vi "PC_HMI_Lift.vi"() -> ()   [LabVIEW 2014]
panel:
  out "Boolean 12":bool
  out "Boolean 11":bool
  out "Boolean 10":bool
  out "Boolean 9":bool
  out "Boolean 8":bool
  out "Boolean 7":bool
  out "Boolean 6":bool
  out "Boolean 5":bool
  out "Boolean 4":bool
  out "Boolean 3":bool
  out "Boolean 2":bool
  out "Boolean":bool
  out "6":bool
  out "4":bool
  out "5":bool
  out "3":bool
  out "2":bool
  out "1":bool
  out "0":bool
  in  "STOP":bool
  in  "SPRAT 5":bool
  in  "SPRAT 4":bool
  in  "SPRAT 3":bool
  in  "SPRAT 2":bool
  in  "SPRAT 1":bool
  in  "SPRAT 0":bool
  out "IDLE":bool
  out "SHUTDOWN":bool
  out "MOVING":bool
  out "DOOR OPEN":bool
  in  "GORE 4":bool
  in  "DOLE 4":bool
  in  "DOLE 5":bool
  in  "GORE 3":bool
  in  "DOLE 3":bool
  in  "GORE 2":bool
  in  "DOLE 2":bool
  in  "GORE 1":bool
  in  "DOLE 1":bool
  in  "GORE 0":bool
  out "Meter":dbl(knob) scale=0.0..5.0
  out "x":dbl
  out "GRAFIK":dbl(graph)
  out "u":dbl
  # "SPRAT 5"
  # "SPRAT 4"
  # "SPRAT 3"
  # "SPRAT 2"
  # "SPRAT 1"
  # "PRIZEMLJE"
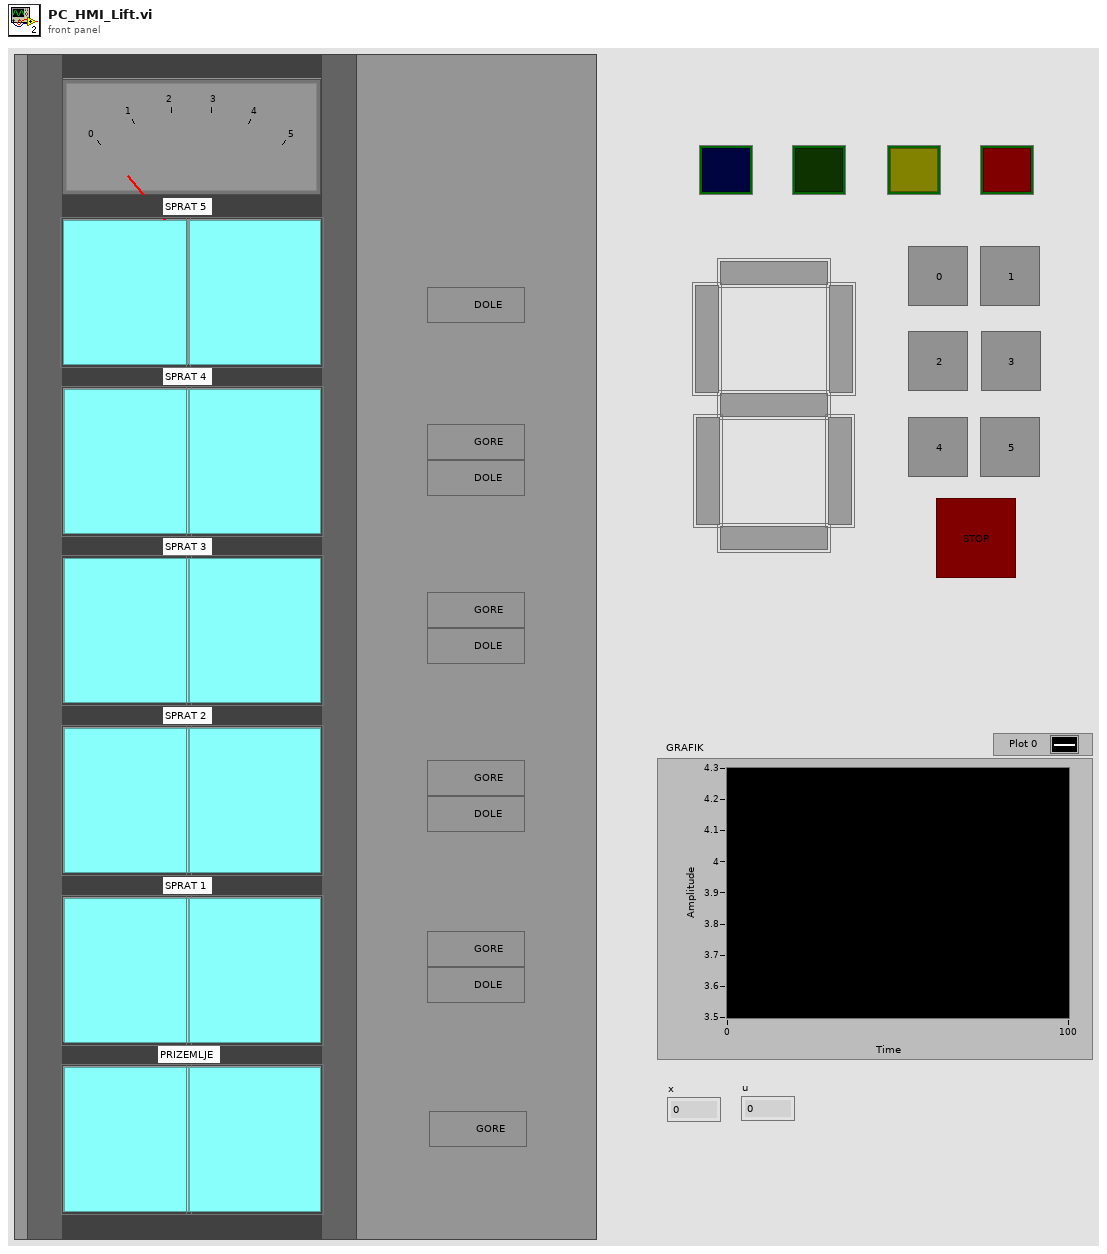
[diagram p1: front panel]
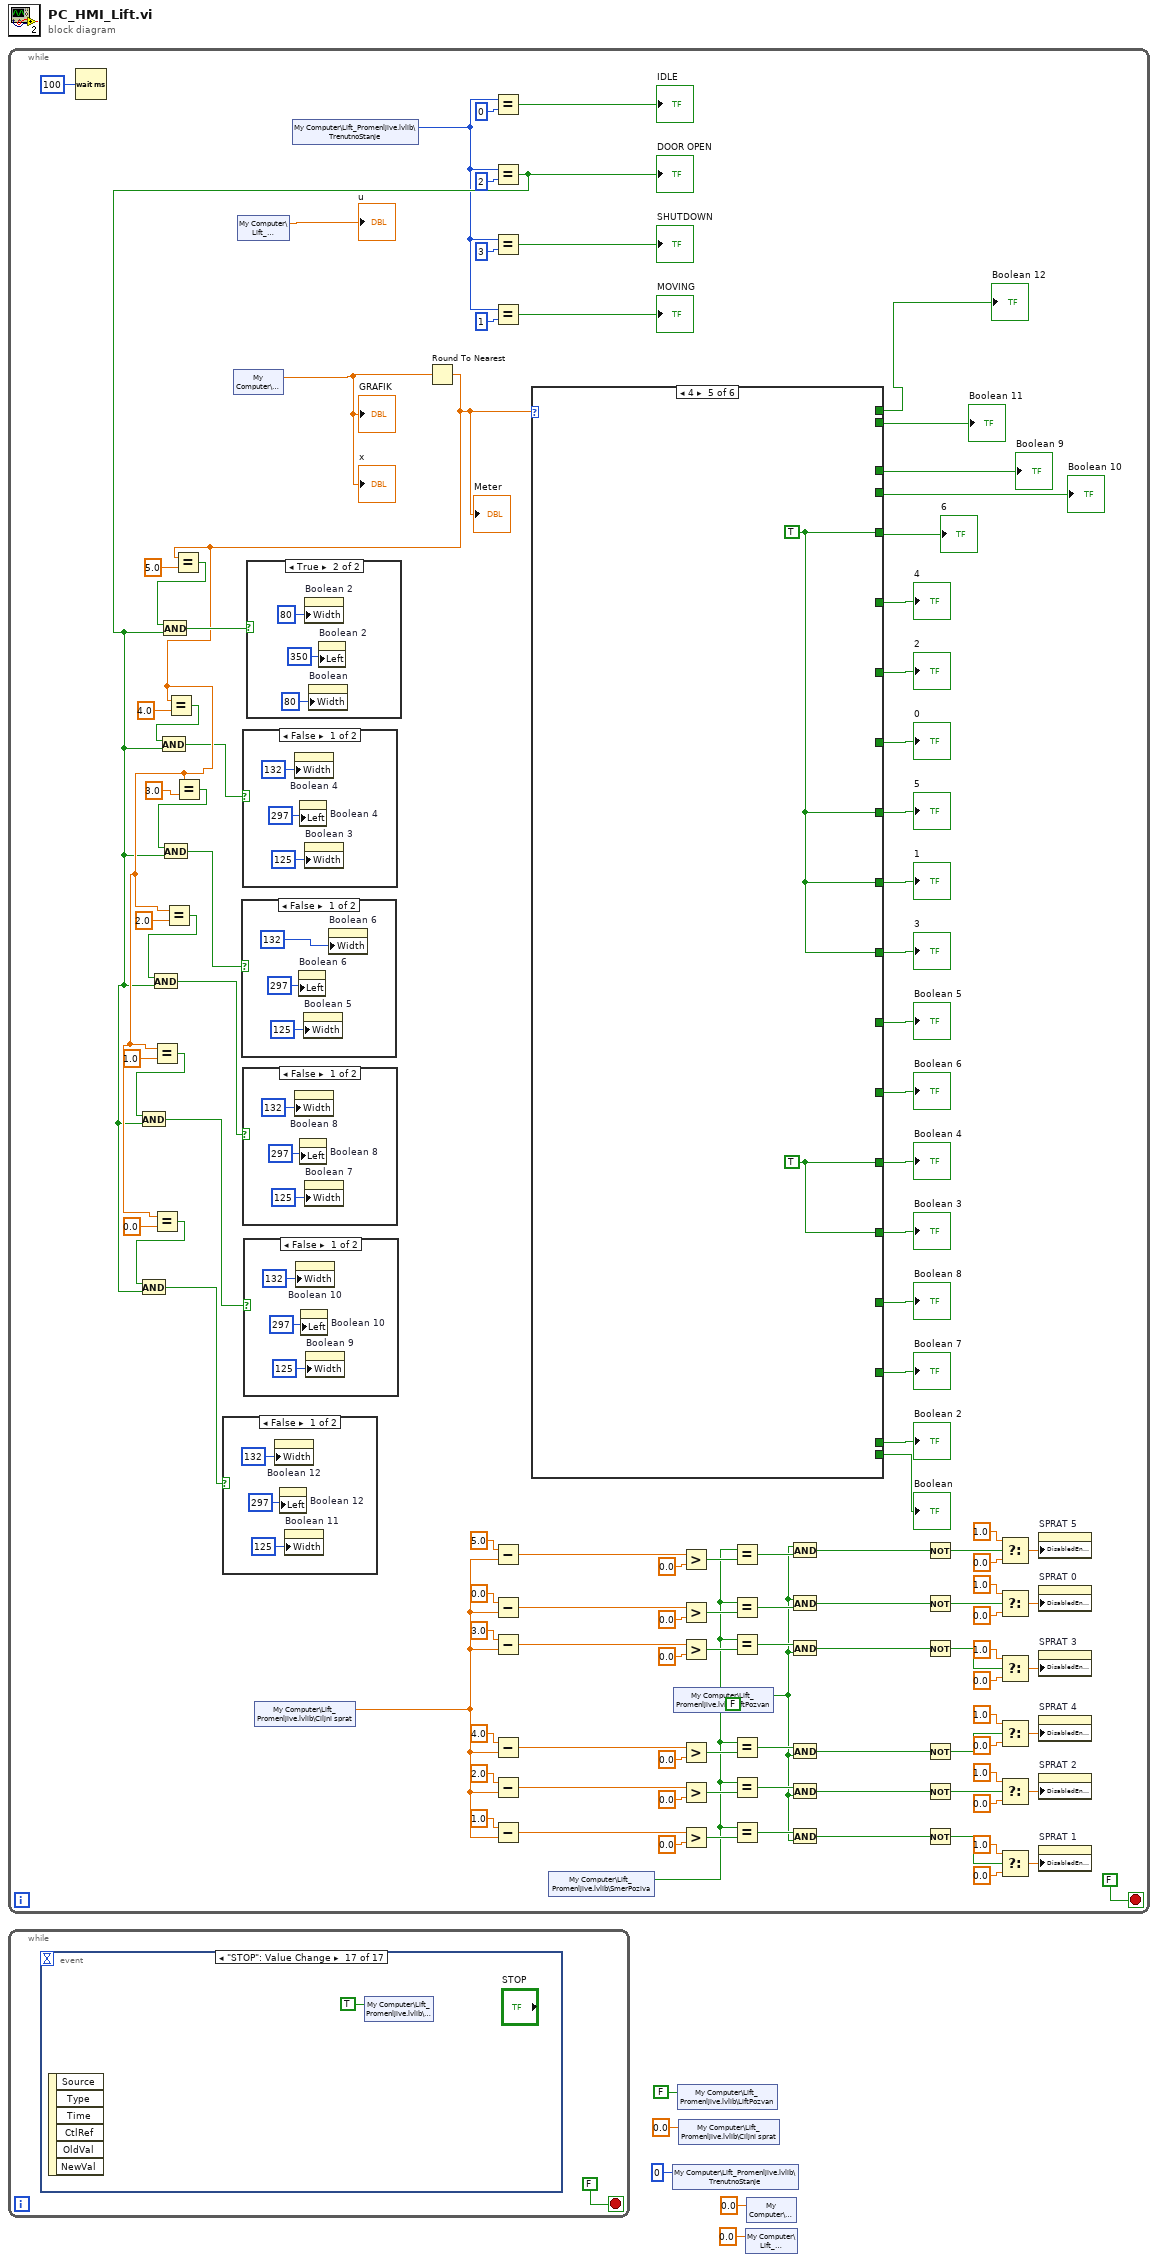
[diagram p0: block diagram]
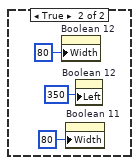
[diagram p2: hidden frame]
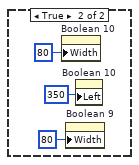
[diagram p3: hidden frame]
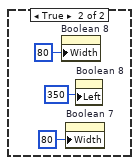
[diagram p4: hidden frame]
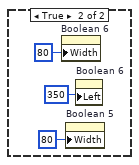
[diagram p5: hidden frame]
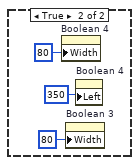
[diagram p6: hidden frame]
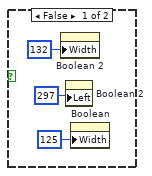
[diagram p7: hidden frame]
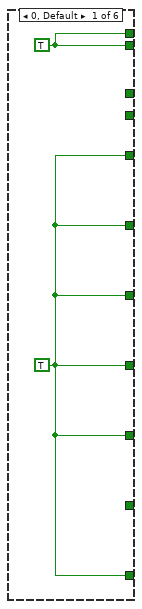
[diagram p8: hidden frame]
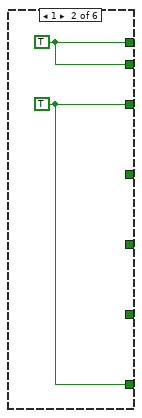
[diagram p9: hidden frame]
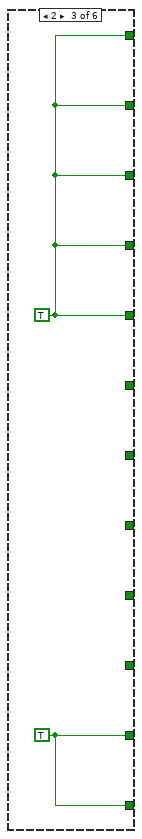
[diagram p10: hidden frame]
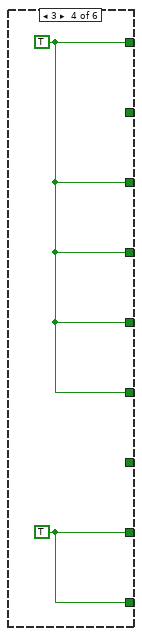
[diagram p11: hidden frame]
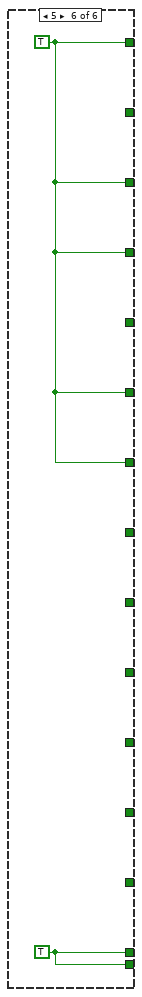
[diagram p12: hidden frame]
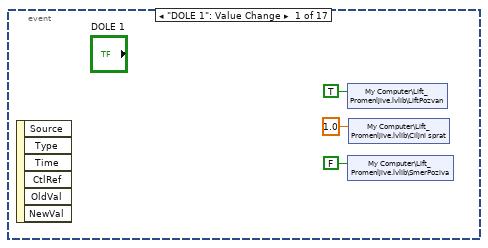
[diagram p13: hidden frame]
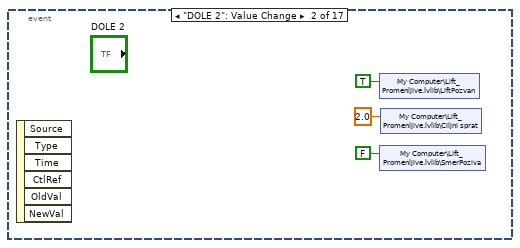
[diagram p14: hidden frame]
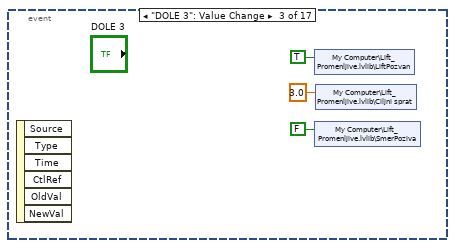
[diagram p15: hidden frame]
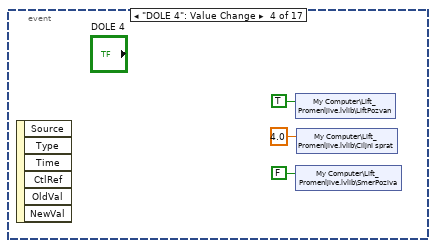
[diagram p16: hidden frame]
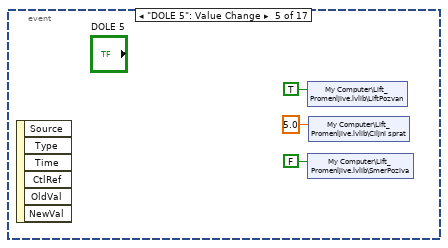
[diagram p17: hidden frame]
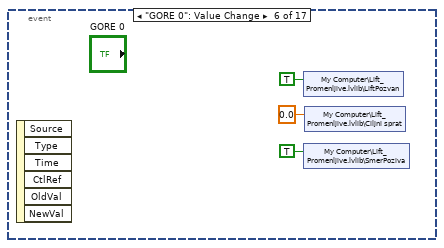
[diagram p18: hidden frame]
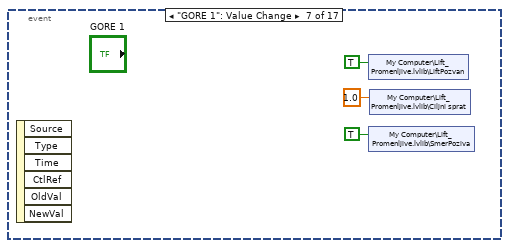
[diagram p19: hidden frame]
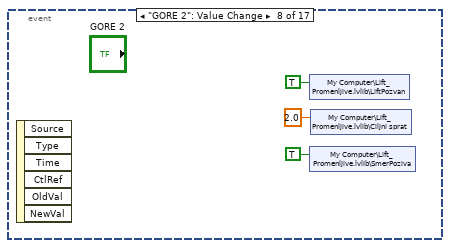
[diagram p20: hidden frame]
diagram:
  n1 = while {
    stop <- FALSE stop-if-true
    (unwired) FALSE
    n2 = Wait (ms)(milliseconds to wait=u32 100) -> ()  [unwired: 1 out]
    n3 = shared-variable "My Computer\\Lift_Promenljive.lvlib\\x"() -> (w9:dbl)  [unwired: 1 in, 1 out]
    "x" <- w9
    "GRAFIK" <- w9
    n4 = shared-variable "My Computer\\Lift_Promenljive.lvlib\\u"() -> (→"u":dbl)  [unwired: 1 in, 1 out]
    n5 = shared-variable "My Computer\\Lift_Promenljive.lvlib\\Ciljni sprat"() -> (w7:dbl)  [unwired: 1 in, 1 out]
    n6 = shared-variable "My Computer\\Lift_Promenljive.lvlib\\TrenutnoStanje"() -> (w11:u8)  [unwired: 1 in, 1 out]
    n7 = Round To Nearest(number=w9) -> (nearest integer value=w18:dbl)
    "Meter" <- w18
    n8 = Equal?(x=w18, y=1.0) -> (x = y?=w21:bool)
    n9 = Equal?(x=w18, y=0.0) -> (x = y?=w19:bool)
    n10 = Equal?(x=w18, y=2.0) -> (x = y?=w23:bool)
    n11 = Equal?(x=w18, y=4.0) -> (x = y?=w27:bool)
    n12 = Equal?(x=w18, y=5.0) -> (x = y?=w30:bool)
    n13 = Equal?(x=w18, y=3.0) -> (x = y?=w25:bool)
    n14 = Equal?(x=w11, y=0) -> (x = y?=→"IDLE":bool)
    n15 = Equal?(x=w11, y=2) -> (x = y?=w17:bool)
    "DOOR OPEN" <- w17
    n16 = And(x=w21, y=w17) -> (x .and. y?=w15:bool)
    n17 = And(x=w19, y=w17) -> (x .and. y?=w16:bool)
    n18 = And(x=w23, y=w17) -> (x .and. y?=w14:bool)
    n19 = And(x=w27, y=w17) -> (x .and. y?=w12:bool)
    n20 = And(x=w30, y=w17) -> (x .and. y?=w29:bool)
    n21 = And(x=w25, y=w17) -> (x .and. y?=w13:bool)
    n22 = case shown="False" w16 {
      frame False {
        n23 = property on="Boolean 12" class="Bool (strict)"("Width"=u32 132 ("Button Size:Width")) -> ()  [unwired: 2 in, 2 out]
        n24 = property on="Boolean 12" class="Bool (strict)"("Left"=297 ("Position:Left")) -> ()  [unwired: 2 in, 2 out]
        n25 = property on="Boolean 11" class="Bool (strict)"("Width"=u32 125 ("Button Size:Width")) -> ()  [unwired: 2 in, 2 out]
      }
      frame True {
        n26 = property on="Boolean 12" class="Bool (strict)"("Width"=u32 80 ("Button Size:Width")) -> ()  [unwired: 2 in, 2 out]
        n27 = property on="Boolean 11" class="Bool (strict)"("Width"=u32 80 ("Button Size:Width")) -> ()  [unwired: 2 in, 2 out]
        n28 = property on="Boolean 12" class="Bool (strict)"("Left"=350 ("Position:Left")) -> ()  [unwired: 2 in, 2 out]
      }
    }
    n29 = case shown="False" w13 {
      frame False {
        n30 = property on="Boolean 6" class="Bool (strict)"("Left"=297 ("Position:Left")) -> ()  [unwired: 2 in, 2 out]
        n31 = property on="Boolean 5" class="Bool (strict)"("Width"=u32 125 ("Button Size:Width")) -> ()  [unwired: 2 in, 2 out]
        n32 = property on="Boolean 6" class="Bool (strict)"("Width"=u32 132 ("Button Size:Width")) -> ()  [unwired: 2 in, 2 out]
      }
      frame True {
        n33 = property on="Boolean 6" class="Bool (strict)"("Width"=u32 80 ("Button Size:Width")) -> ()  [unwired: 2 in, 2 out]
        n34 = property on="Boolean 5" class="Bool (strict)"("Width"=u32 80 ("Button Size:Width")) -> ()  [unwired: 2 in, 2 out]
        n35 = property on="Boolean 6" class="Bool (strict)"("Left"=350 ("Position:Left")) -> ()  [unwired: 2 in, 2 out]
      }
    }
    n36 = case shown="False" w12 {
      frame False {
        n37 = property on="Boolean 4" class="Bool (strict)"("Width"=u32 132 ("Button Size:Width")) -> ()  [unwired: 2 in, 2 out]
        n38 = property on="Boolean 4" class="Bool (strict)"("Left"=297 ("Position:Left")) -> ()  [unwired: 2 in, 2 out]
        n39 = property on="Boolean 3" class="Bool (strict)"("Width"=u32 125 ("Button Size:Width")) -> ()  [unwired: 2 in, 2 out]
      }
      frame True {
        n40 = property on="Boolean 4" class="Bool (strict)"("Width"=u32 80 ("Button Size:Width")) -> ()  [unwired: 2 in, 2 out]
        n41 = property on="Boolean 3" class="Bool (strict)"("Width"=u32 80 ("Button Size:Width")) -> ()  [unwired: 2 in, 2 out]
        n42 = property on="Boolean 4" class="Bool (strict)"("Left"=350 ("Position:Left")) -> ()  [unwired: 2 in, 2 out]
      }
    }
    n43 = case shown="False" w14 {
      frame False {
        n44 = property on="Boolean 8" class="Bool (strict)"("Width"=u32 132 ("Button Size:Width")) -> ()  [unwired: 2 in, 2 out]
        n45 = property on="Boolean 8" class="Bool (strict)"("Left"=297 ("Position:Left")) -> ()  [unwired: 2 in, 2 out]
        n46 = property on="Boolean 7" class="Bool (strict)"("Width"=u32 125 ("Button Size:Width")) -> ()  [unwired: 2 in, 2 out]
      }
      frame True {
        n47 = property on="Boolean 8" class="Bool (strict)"("Width"=u32 80 ("Button Size:Width")) -> ()  [unwired: 2 in, 2 out]
        n48 = property on="Boolean 7" class="Bool (strict)"("Width"=u32 80 ("Button Size:Width")) -> ()  [unwired: 2 in, 2 out]
        n49 = property on="Boolean 8" class="Bool (strict)"("Left"=350 ("Position:Left")) -> ()  [unwired: 2 in, 2 out]
      }
    }
    n50 = case shown="False" w15 {
      frame False {
        n51 = property on="Boolean 10" class="Bool (strict)"("Width"=u32 132 ("Button Size:Width")) -> ()  [unwired: 2 in, 2 out]
        n52 = property on="Boolean 10" class="Bool (strict)"("Left"=297 ("Position:Left")) -> ()  [unwired: 2 in, 2 out]
        n53 = property on="Boolean 9" class="Bool (strict)"("Width"=u32 125 ("Button Size:Width")) -> ()  [unwired: 2 in, 2 out]
      }
      frame True {
        n54 = property on="Boolean 10" class="Bool (strict)"("Width"=u32 80 ("Button Size:Width")) -> ()  [unwired: 2 in, 2 out]
        n55 = property on="Boolean 9" class="Bool (strict)"("Width"=u32 80 ("Button Size:Width")) -> ()  [unwired: 2 in, 2 out]
        n56 = property on="Boolean 10" class="Bool (strict)"("Left"=350 ("Position:Left")) -> ()  [unwired: 2 in, 2 out]
      }
    }
    n57 = case shown="True" w29 {
      frame False {
        n58 = property on="Boolean 2" class="Bool (strict)"("Width"=u32 132 ("Button Size:Width")) -> ()  [unwired: 2 in, 2 out]
        n59 = property on="Boolean 2" class="Bool (strict)"("Left"=297 ("Position:Left")) -> ()  [unwired: 2 in, 2 out]
        n60 = property on="Boolean" class="Bool (strict)"("Width"=u32 125 ("Button Size:Width")) -> ()  [unwired: 2 in, 2 out]
      }
      frame True {
        n61 = property on="Boolean 2" class="Bool (strict)"("Width"=u32 80 ("Button Size:Width")) -> ()  [unwired: 2 in, 2 out]
        n62 = property on="Boolean" class="Bool (strict)"("Width"=u32 80 ("Button Size:Width")) -> ()  [unwired: 2 in, 2 out]
        n63 = property on="Boolean 2" class="Bool (strict)"("Left"=350 ("Position:Left")) -> ()  [unwired: 2 in, 2 out]
      }
    }
    n64 = Equal?(x=w11, y=3) -> (x = y?=→"SHUTDOWN":bool)
    n65 = Equal?(x=w11, y=1) -> (x = y?=→"MOVING":bool)
    n66 = Subtract(x=5.0, y=w7) -> (x-y=w59:dbl)
    n67 = Subtract(x=0.0 ("y"), y=w7) -> (x-y=w68:dbl)
    n68 = Subtract(x=3.0 ("y"), y=w7) -> (x-y=w100:dbl)
    n69 = Subtract(x=4.0 ("y"), y=w7) -> (x-y=w99:dbl)
    n70 = Subtract(x=2.0 ("y"), y=w7) -> (x-y=w101:dbl)
    n71 = Subtract(x=1.0 ("y"), y=w7) -> (x-y=w105:dbl)
    n72 = case shown="4" w18 {
      tunnel: [w157 _ w161 w163 _ w167] -> w32
      tunnel: [_ _ w161 w163 w165 w167] -> w33
      tunnel: [w157 _ w161 w163 _ w167] -> w34
      tunnel: [w157 _ _ _ w165 w167] -> w35
      tunnel: [w157 _ w161 _ _ _] -> w36
      tunnel: [w157 w159 _ w163 w165 w167] -> w37
      tunnel: [w157 w159 w161 w163 w165 _] -> w38
      tunnel: [w156 _ _ _ _ _] -> w39
      tunnel: [w156 _ _ _ _ _] -> w40
      tunnel: [_ w158 _ _ _ _] -> w41
      tunnel: [_ w158 _ _ _ _] -> w42
      tunnel: [_ _ w160 _ _ _] -> w43
      tunnel: [_ _ w160 _ _ _] -> w44
      tunnel: [_ _ _ w162 _ _] -> w45
      tunnel: [_ _ _ w162 _ _] -> w46
      tunnel: [_ _ _ _ w164 _] -> w47
      tunnel: [_ _ _ _ w164 _] -> w48
      tunnel: [_ _ _ _ _ w166] -> w49
      tunnel: [_ _ _ _ _ w166] -> w50
      frame 0, Default {
        w156 = TRUE
        w157 = TRUE
      }
      frame 1 {
        w158 = TRUE
        w159 = TRUE
      }
      frame 2 {
        w160 = TRUE
        w161 = TRUE
      }
      frame 3 {
        w162 = TRUE
        w163 = TRUE
      }
      frame 4 {
        w164 = TRUE
        w165 = TRUE
      }
      frame 5 {
        w166 = TRUE
        w167 = TRUE
      }
    }
    "1" <- w33
    "2" <- w34
    "3" <- w35
    "5" <- w38
    "4" <- w36
    "6" <- w37
    "0" <- w32
    "Boolean 2" <- w50
    "Boolean" <- w49
    "Boolean 3" <- w48
    "Boolean 4" <- w47
    "Boolean 5" <- w45
    "Boolean 7" <- w43
    "Boolean 6" <- w46
    "Boolean 12" <- w40
    "Boolean 8" <- w44
    "Boolean 10" <- w42
    "Boolean 9" <- w41
    "Boolean 11" <- w39
    n73 = shared-variable "My Computer\\Lift_Promenljive.lvlib\\SmerPoziva"() -> (w6:bool)  [unwired: 1 in, 1 out]
    n74 = shared-variable "My Computer\\Lift_Promenljive.lvlib\\LiftPozvan"() -> (w8:bool)  [unwired: 1 in, 1 out]
    n75 = Greater?(x=w59, y=0.0) -> (0:w57:bool)
    n76 = Greater?(x=w68, y=0.0) -> (0:w67:bool)
    n77 = Greater?(x=w100, y=0.0) -> (0:w96:bool)
    n78 = Greater?(x=w99, y=0.0) -> (0:w95:bool)
    n79 = Greater?(x=w101, y=0.0) -> (0:w97:bool)
    n80 = Greater?(x=w105, y=0.0) -> (0:w98:bool)
    n81 = Equal?(x=w6, y=w57) -> (x = y?=w56:bool)
    n82 = Equal?(x=w6, y=w67) -> (x = y?=w66:bool)
    n83 = Equal?(x=w6, y=w96) -> (x = y?=w92:bool)
    n84 = Equal?(x=w6, y=w95) -> (x = y?=w91:bool)
    n85 = Equal?(x=w6, y=w97) -> (x = y?=w93:bool)
    n86 = Equal?(x=w6, y=w98) -> (x = y?=w94:bool)
    n87 = And(x=w8, y=w56) -> (x .and. y?=w55:bool)
    n88 = And(x=w8, y=w66) -> (x .and. y?=w65:bool)
    n89 = And(x=w92, y=w8) -> (x .and. y?=w88:bool)
    n90 = And(x=w91, y=w8) -> (x .and. y?=w87:bool)
    n91 = And(x=w93, y=w8) -> (x .and. y?=w89:bool)
    n92 = And(x=w94, y=w8) -> (x .and. y?=w90:bool)
    n93 = Not(x=w55) -> (.not. x?=w52:bool)
    n94 = Not(x=w65) -> (.not. x?=w62:bool)
    n95 = Not(x=w88) -> (.not. x?=w75:bool)
    n96 = Not(x=w87) -> (.not. x?=w74:bool)
    n97 = Not(x=w89) -> (.not. x?=w76:bool)
    n98 = Not(x=w90) -> (.not. x?=w86:bool)
    n99 = Select(t=1.0, s=w52, f=0.0) -> (s? t:f=w51:dbl)
    n100 = Select(t=1.0, s=w62, f=0.0) -> (s? t:f=w61:dbl)
    n101 = Select(t=1.0, s=w75, f=0.0) -> (s? t:f=w72:dbl)
    n102 = Select(t=1.0, s=w74, f=0.0) -> (s? t:f=w71:dbl)
    n103 = Select(t=1.0, s=w76, f=0.0) -> (s? t:f=w73:dbl)
    n104 = Select(t=1.0, s=w86, f=0.0) -> (s? t:f=w83:dbl)
    n105 = property on="SPRAT 5" class="Bool"("DisabledEnum"=w51) -> ()  [unwired: 2 in, 2 out]
    n106 = property on="SPRAT 0" class="Bool"("DisabledEnum"=w61) -> ()  [unwired: 2 in, 2 out]
    n107 = property on="SPRAT 3" class="Bool"("DisabledEnum"=w72) -> ()  [unwired: 2 in, 2 out]
    n108 = property on="SPRAT 4" class="Bool"("DisabledEnum"=w71) -> ()  [unwired: 2 in, 2 out]
    n109 = property on="SPRAT 2" class="Bool"("DisabledEnum"=w73) -> ()  [unwired: 2 in, 2 out]
    n110 = property on="SPRAT 1" class="Bool"("DisabledEnum"=w83) -> ()  [unwired: 2 in, 2 out]
  }
  n111 = while {
    stop <- FALSE stop-if-true
    n112 = event shown="[16] \"STOP\": Value Change" {
      selector: _ -> [_ _ _ _ _ _ _ _ _ _ _ _ _ _ _ _ _]
      dyn-events: _ -> [_ _ _ _ _ _ _ _ _ _ _ _ _ _ _ _ _]
      timeout: _ -> [_ _ _ _ _ _ _ _ _ _ _ _ _ _ _ _ _]
      event "DOLE 1": Value Change {
        n113 = event-data() -> ()  [unwired: 1 in, 6 out]
        n114 = shared-variable "My Computer\\Lift_Promenljive.lvlib\\LiftPozvan"(TRUE ("LiftPozvan")) -> ()  [unwired: 1 in, 1 out]
        n115 = shared-variable "My Computer\\Lift_Promenljive.lvlib\\SmerPoziva"(FALSE ("SmerPoziva")) -> ()  [unwired: 1 in, 1 out]
        n116 = shared-variable "My Computer\\Lift_Promenljive.lvlib\\Ciljni sprat"(1.0 ("Ciljni sprat")) -> ()  [unwired: 1 in, 1 out]
      }
      event "DOLE 2": Value Change {
        n117 = event-data() -> ()  [unwired: 1 in, 6 out]
        n118 = shared-variable "My Computer\\Lift_Promenljive.lvlib\\LiftPozvan"(TRUE ("LiftPozvan")) -> ()  [unwired: 1 in, 1 out]
        n119 = shared-variable "My Computer\\Lift_Promenljive.lvlib\\SmerPoziva"(FALSE ("SmerPoziva")) -> ()  [unwired: 1 in, 1 out]
        n120 = shared-variable "My Computer\\Lift_Promenljive.lvlib\\Ciljni sprat"(2.0 ("Ciljni sprat")) -> ()  [unwired: 1 in, 1 out]
      }
      event "DOLE 3": Value Change {
        n121 = event-data() -> ()  [unwired: 1 in, 6 out]
        n122 = shared-variable "My Computer\\Lift_Promenljive.lvlib\\LiftPozvan"(TRUE ("LiftPozvan")) -> ()  [unwired: 1 in, 1 out]
        n123 = shared-variable "My Computer\\Lift_Promenljive.lvlib\\SmerPoziva"(FALSE ("SmerPoziva")) -> ()  [unwired: 1 in, 1 out]
        n124 = shared-variable "My Computer\\Lift_Promenljive.lvlib\\Ciljni sprat"(3.0 ("Ciljni sprat")) -> ()  [unwired: 1 in, 1 out]
      }
      event "DOLE 4": Value Change {
        n125 = event-data() -> ()  [unwired: 1 in, 6 out]
        n126 = shared-variable "My Computer\\Lift_Promenljive.lvlib\\LiftPozvan"(TRUE ("LiftPozvan")) -> ()  [unwired: 1 in, 1 out]
        n127 = shared-variable "My Computer\\Lift_Promenljive.lvlib\\SmerPoziva"(FALSE ("SmerPoziva")) -> ()  [unwired: 1 in, 1 out]
        n128 = shared-variable "My Computer\\Lift_Promenljive.lvlib\\Ciljni sprat"(4.0 ("Ciljni sprat")) -> ()  [unwired: 1 in, 1 out]
      }
      event "DOLE 5": Value Change {
        n129 = event-data() -> ()  [unwired: 1 in, 6 out]
        n130 = shared-variable "My Computer\\Lift_Promenljive.lvlib\\LiftPozvan"(TRUE ("LiftPozvan")) -> ()  [unwired: 1 in, 1 out]
        n131 = shared-variable "My Computer\\Lift_Promenljive.lvlib\\SmerPoziva"(FALSE ("SmerPoziva")) -> ()  [unwired: 1 in, 1 out]
        n132 = shared-variable "My Computer\\Lift_Promenljive.lvlib\\Ciljni sprat"(5.0 ("Ciljni sprat")) -> ()  [unwired: 1 in, 1 out]
      }
      event "GORE 0": Value Change {
        n133 = event-data() -> ()  [unwired: 1 in, 6 out]
        n134 = shared-variable "My Computer\\Lift_Promenljive.lvlib\\LiftPozvan"(TRUE ("LiftPozvan")) -> ()  [unwired: 1 in, 1 out]
        n135 = shared-variable "My Computer\\Lift_Promenljive.lvlib\\SmerPoziva"(TRUE ("SmerPoziva")) -> ()  [unwired: 1 in, 1 out]
        n136 = shared-variable "My Computer\\Lift_Promenljive.lvlib\\Ciljni sprat"(0.0 ("Ciljni sprat")) -> ()  [unwired: 1 in, 1 out]
      }
      event "GORE 1": Value Change {
        n137 = event-data() -> ()  [unwired: 1 in, 6 out]
        n138 = shared-variable "My Computer\\Lift_Promenljive.lvlib\\LiftPozvan"(TRUE ("LiftPozvan")) -> ()  [unwired: 1 in, 1 out]
        n139 = shared-variable "My Computer\\Lift_Promenljive.lvlib\\SmerPoziva"(TRUE ("SmerPoziva")) -> ()  [unwired: 1 in, 1 out]
        n140 = shared-variable "My Computer\\Lift_Promenljive.lvlib\\Ciljni sprat"(1.0 ("Ciljni sprat")) -> ()  [unwired: 1 in, 1 out]
      }
      event "GORE 2": Value Change {
        n141 = event-data() -> ()  [unwired: 1 in, 6 out]
        n142 = shared-variable "My Computer\\Lift_Promenljive.lvlib\\LiftPozvan"(TRUE ("LiftPozvan")) -> ()  [unwired: 1 in, 1 out]
        n143 = shared-variable "My Computer\\Lift_Promenljive.lvlib\\SmerPoziva"(TRUE ("SmerPoziva")) -> ()  [unwired: 1 in, 1 out]
        n144 = shared-variable "My Computer\\Lift_Promenljive.lvlib\\Ciljni sprat"(2.0 ("Ciljni sprat")) -> ()  [unwired: 1 in, 1 out]
      }
      event "GORE 3": Value Change {
        n145 = event-data() -> ()  [unwired: 1 in, 6 out]
        n146 = shared-variable "My Computer\\Lift_Promenljive.lvlib\\LiftPozvan"(TRUE ("LiftPozvan")) -> ()  [unwired: 1 in, 1 out]
        n147 = shared-variable "My Computer\\Lift_Promenljive.lvlib\\SmerPoziva"(TRUE ("SmerPoziva")) -> ()  [unwired: 1 in, 1 out]
        n148 = shared-variable "My Computer\\Lift_Promenljive.lvlib\\Ciljni sprat"(3.0 ("Ciljni sprat")) -> ()  [unwired: 1 in, 1 out]
      }
      event "GORE 4": Value Change {
        n149 = event-data() -> ()  [unwired: 1 in, 6 out]
        n150 = shared-variable "My Computer\\Lift_Promenljive.lvlib\\LiftPozvan"(TRUE ("LiftPozvan")) -> ()  [unwired: 1 in, 1 out]
        n151 = shared-variable "My Computer\\Lift_Promenljive.lvlib\\SmerPoziva"(TRUE ("SmerPoziva")) -> ()  [unwired: 1 in, 1 out]
        n152 = shared-variable "My Computer\\Lift_Promenljive.lvlib\\Ciljni sprat"(4.0 ("Ciljni sprat")) -> ()  [unwired: 1 in, 1 out]
      }
      event "SPRAT 0": Value Change {
        n153 = event-data() -> ()  [unwired: 1 in, 6 out]
        n154 = shared-variable "My Computer\\Lift_Promenljive.lvlib\\Ciljni sprat"(0.0 ("Ciljni sprat")) -> ()  [unwired: 1 in, 1 out]
        n155 = shared-variable "My Computer\\Lift_Promenljive.lvlib\\LiftPozvan"(FALSE ("LiftPozvan")) -> ()  [unwired: 1 in, 1 out]
      }
      event "SPRAT 1": Value Change {
        n156 = event-data() -> ()  [unwired: 1 in, 6 out]
        n157 = shared-variable "My Computer\\Lift_Promenljive.lvlib\\Ciljni sprat"(1.0 ("Ciljni sprat")) -> ()  [unwired: 1 in, 1 out]
        n158 = shared-variable "My Computer\\Lift_Promenljive.lvlib\\LiftPozvan"(FALSE ("LiftPozvan")) -> ()  [unwired: 1 in, 1 out]
      }
      event "SPRAT 2": Value Change {
        n159 = event-data() -> ()  [unwired: 1 in, 6 out]
        n160 = shared-variable "My Computer\\Lift_Promenljive.lvlib\\Ciljni sprat"(2.0 ("Ciljni sprat")) -> ()  [unwired: 1 in, 1 out]
        n161 = shared-variable "My Computer\\Lift_Promenljive.lvlib\\LiftPozvan"(FALSE ("LiftPozvan")) -> ()  [unwired: 1 in, 1 out]
      }
      event "SPRAT 3": Value Change {
        n162 = event-data() -> ()  [unwired: 1 in, 6 out]
        n163 = shared-variable "My Computer\\Lift_Promenljive.lvlib\\Ciljni sprat"(3.0 ("Ciljni sprat")) -> ()  [unwired: 1 in, 1 out]
        n164 = shared-variable "My Computer\\Lift_Promenljive.lvlib\\LiftPozvan"(FALSE ("LiftPozvan")) -> ()  [unwired: 1 in, 1 out]
      }
      event "SPRAT 4": Value Change {
        n165 = event-data() -> ()  [unwired: 1 in, 6 out]
        n166 = shared-variable "My Computer\\Lift_Promenljive.lvlib\\Ciljni sprat"(4.0 ("Ciljni sprat")) -> ()  [unwired: 1 in, 1 out]
        n167 = shared-variable "My Computer\\Lift_Promenljive.lvlib\\LiftPozvan"(FALSE ("LiftPozvan")) -> ()  [unwired: 1 in, 1 out]
      }
      event "SPRAT 5": Value Change {
        n168 = event-data() -> ()  [unwired: 1 in, 6 out]
        n169 = shared-variable "My Computer\\Lift_Promenljive.lvlib\\Ciljni sprat"(5.0 ("Ciljni sprat")) -> ()  [unwired: 1 in, 1 out]
        n170 = shared-variable "My Computer\\Lift_Promenljive.lvlib\\LiftPozvan"(FALSE ("LiftPozvan")) -> ()  [unwired: 1 in, 1 out]
      }
      event "STOP": Value Change {
        n171 = event-data() -> ()  [unwired: 1 in, 6 out]
        n172 = shared-variable "My Computer\\Lift_Promenljive.lvlib\\Stop"(TRUE ("Stop")) -> ()  [unwired: 1 in, 1 out]
      }
    }
  }
  n173 = shared-variable "My Computer\\Lift_Promenljive.lvlib\\TrenutnoStanje"(u8 0 ("TrenutnoStanje")) -> ()  [unwired: 1 in, 1 out]
  n174 = shared-variable "My Computer\\Lift_Promenljive.lvlib\\LiftPozvan"(FALSE ("LiftPozvan")) -> ()  [unwired: 1 in, 1 out]
  n175 = shared-variable "My Computer\\Lift_Promenljive.lvlib\\Ciljni sprat"(0.0 ("Ciljni sprat")) -> ()  [unwired: 1 in, 1 out]
  n176 = shared-variable "My Computer\\Lift_Promenljive.lvlib\\u"(0.0 ("u")) -> ()  [unwired: 1 in, 1 out]
  n177 = shared-variable "My Computer\\Lift_Promenljive.lvlib\\x"(0.0 ("x")) -> ()  [unwired: 1 in, 1 out]
